vi "FGV-StatusChangeEventRef.vi"(8 "error in (no error)":errorcluster, 11 "Name(\"\" to use uuid) in":string) -> (0 "error out":errorcluster, 3 "Status Change Event":refnum<user-event>)   [LabVIEW 2017, in "Communicable State Machine.lvlib"]
doc: "-- <b>Controls</b> --\n- <b>Name(\"\" to use uuid) in</b>:\n\n-- <b>Indicators</b> --\n- <b>Status Change Event</b>:"
uses:
  Communicable State Machine.lvlib
  Typedef/_CSM Status Change Event Data.ctl
  CSMQ/_CSMOFGVOPER.ctl
  FGV-BroadcastRegistry/global-CSMQ FGV Change Flag.vi
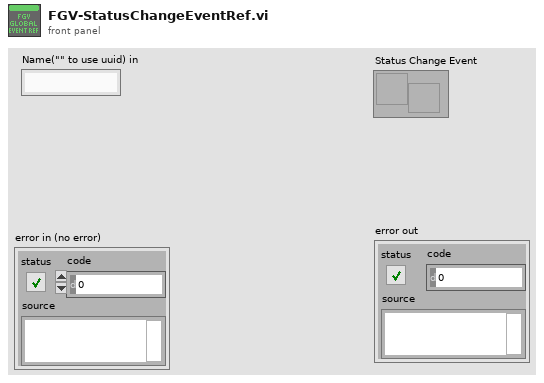
[diagram p1: front panel]
types:
  T1 = typedef "Communicable State Machine.lvlib/_CSMOFGVOPER.ctl" = enum16{"Create If not Exist", "Get By Name", "List", "Check If Name Exists", "Release", "Module Status", "Create Status Event Handler", "Destroy Status Event Handler", "Clear Invalid Objs"}
  T2 = typedef "Communicable State Machine.lvlib/_CSMObj.ctl" = cluster{"info":T3, "Refs":T5}
  T3 = typedef "Communicable State Machine.lvlib/_CSMObj-Info.ctl" = cluster{"Module Name":string, "Requested Name":string, "Group Name":string, "Mode":T4, "Allowed Messages":string[]}
  T4 = typedef "Communicable State Machine.lvlib/_CSM_MODE.ctl" = enum16{"Not Exist", "Stand Alone", "CSM", "Worker", "Worker Agent", "Chain Node", "Chain"}
  T5 = typedef "Communicable State Machine.lvlib/_CSMObj-Refs.ctl" = cluster{"WatchDogQ":refnum<queue>, "CSMDataDVR":refnum<data-value>, "Queue":refnum<class "Priority Queue.lvclass">, "GroupDataDVR":refnum<data-value>, "TagMap":refnum<data-value>, "Exit Event":refnum<user-event>, "NewStateEvent":refnum<user-event>, "StatusChangeEvent":refnum<user-event>}
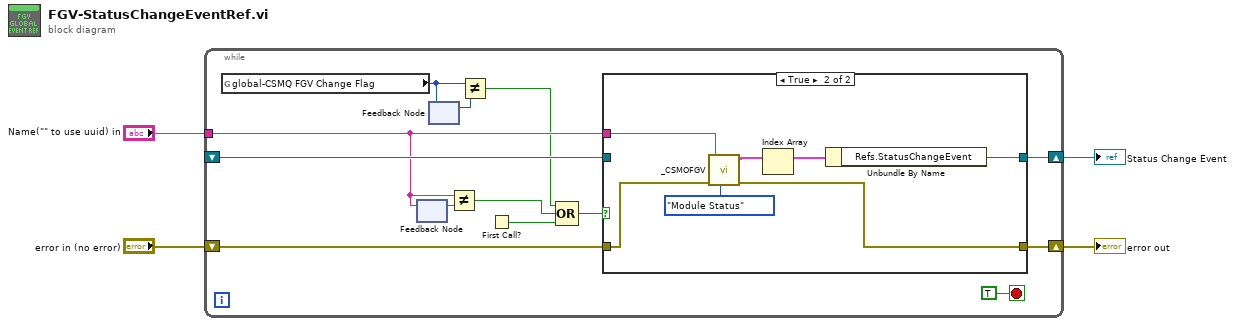
[diagram p0: block diagram]
diagram:
  n1 = while {
    shift-right: [w15] -> w2
    shift-left: "error in (no error)" -> [w16]
    shift-right: [w17] -> w4
    shift-left: _ -> [w13]
    tunnel: "Name(\"\" to use uuid) in" -> [w12]
    stop <- TRUE stop-if-true
    n2 = global read "global-CSMQ FGV Change Flag.vi" "global-CSMQ FGV Change Flag"() -> (w9:u64)
    n3 = feedback-in #1(w12) -> ()
    n4 = feedback #1() -> (w11:string)  [unwired: 1 in]
    n5 = feedback #2() -> (w8:u64)  [unwired: 1 in]
    n6 = feedback-in #2(w9) -> ()
    n7 = Not Equal?(x=w12, y=w11) -> (x != y?=w10:bool)
    n8 = Not Equal?(x=w9, y=w8) -> (x != y?=w5:bool)
    n9 = First Call?() -> (First Call?: T/F=w6:bool)
    n10 = Compound Arithmetic op=OR(w5, w10, w6) -> (w7:bool)
    n11 = case shown="True" w7 {
      tunnel: [w19 w21] -> w17
      tunnel: w16 -> [w18 w24]
      tunnel: [w18 w25] -> w15
      tunnel: w13 -> [w19 _]
      tunnel: w12 -> [_ w20]
      frame False {
      }
      frame True {
        n12 = call "_CSMOFGV.vi"("Operation"=_CSMOFGVOPER."Module Status", "Error in"=w24, "Name(\"\" to use uuid) in"=w20) -> ("Error out"=w25:errorcluster, "Array"=w23:T2[])  [unwired: 6 in, 1 out]
        n13 = Index Array(array=w23) -> (element=w22:T2)  [unwired: 1 in]
        n14 = Unbundle By Name(w22) -> ("Refs.StatusChangeEvent"=w21:refnum<user-event>)
      }
    }
  }
  "Status Change Event" <- w4
  "error out" <- w2
